vi "GetCtlRefsFromVI.vi"(8 "error in":errorcluster, 11 "VI (Caller)":refnum<vi>) -> (0 "error out":errorcluster, 1 "RefArray":refnum<vi>[](array[refnum]), 2 "RefName Array":string[](array[string]), 3 "VI (Caller) Out":refnum<vi>)   [LabVIEW 2020, in "CtlReferences.lvlib" / "CtlReferences.lvclass"]
uses:
  CtlReferences.lvclass
  TypeDefs/ClassID_Enum.ctl
  CtlReferences.lvclass/CtlReferences.ctl
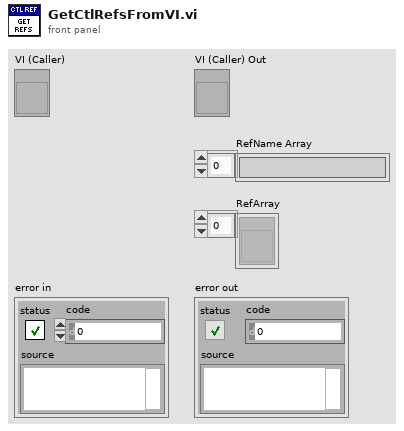
[diagram p1: front panel]
types:
  T1 = typedef "CtlReferences.lvlib/CtlReferences.lvclass/ClassID_Enum.ctl" = enum32{"0 <undefined>", "1 <undefined>", "2 <undefined>", "Generic", "Decoration", "Text", "Control", "ColorBox", "Boolean", "RefNum", "Variant", "Path", "ListBox", "Table", "Array", "Picture", "ActiveXContainer", "Numeric", "Digital", "NamedNumeric", "ColorRamp", "Slide", "GraphOrChart", "WaveformChart", "WaveformGraph", "IntensityChart", "IntensityGraph", "String", "IOName", "ComboBox", "Cluster", "Panel", "Knob", "NumWithScale", "Ring", "Enum", "GObject", "Plot", "Cursor", "NumericText", "Scale", "ColorScale", "GraphScale", "ColorGraphScale", "TypedRefNum", "OldKnobScale", "MCListbox", "MeasureData", "BVTag", "DAQName", "VISAName", "IVIName", "SlideScale", "TabControl", "Page", "TabArrayTabControl", "ConPane"}
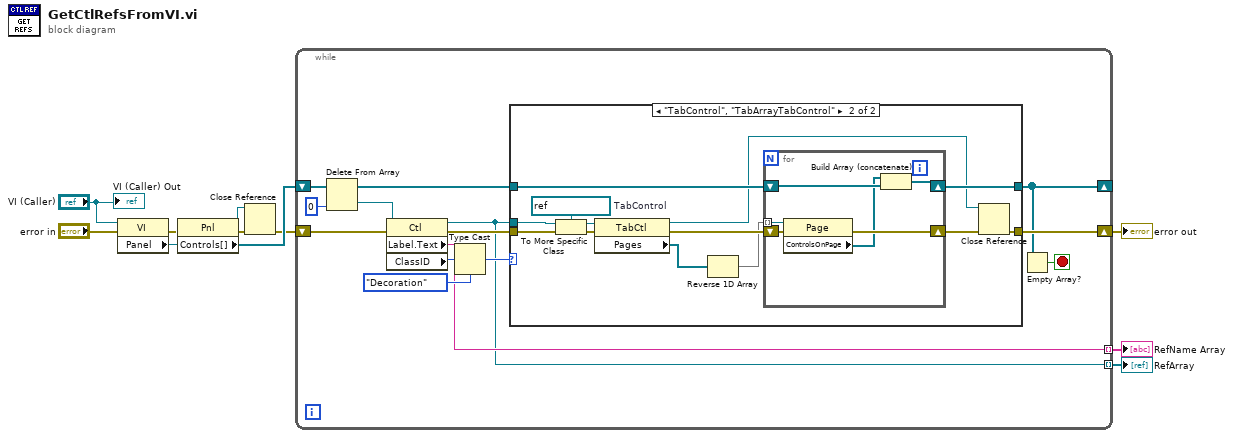
[diagram p0: block diagram]
diagram:
  n1 = property class="VI"(reference="VI (Caller)", error in="error in") -> (error out=w9:errorcluster, "Panel"=w10:refnum<vi>)  [unwired: 1 out]
  n2 = property class="Pnl"(reference=w10, error in=w9) -> (reference out=w6:refnum<vi>, error out=w7:errorcluster, "Controls[]"=w5:refnum<vi>[])
  n3 = Close Reference(reference=w6, error in (no error)=w7) -> (error out=w4:errorcluster)
  n4 = while {
    shift-right: [w21] -> _
    shift-left: w5 -> [w24]
    shift-right: [w25] -> w1
    shift-left: w4 -> [w18]
    tunnel: [w13] -> w3 mode=indexing
    tunnel: [w12] -> w2 mode=indexing
    stop <- w20 stop-if-true
    n5 = Delete From Array(array=w24, index=0) -> (deleted portion=w15:refnum<vi>, array with subset deleted=w22:refnum<vi>[])  [unwired: 1 in]
    n6 = property class="Ctl"(reference=w15, error in=w18) -> (reference out=w12:refnum<vi>, error out=w17:errorcluster, "Label.Text"=w13:string, "ClassID"=w19:u32)
    n7 = Type Cast(type=ClassID_Enum."Decoration" ("ClassID Name"), x=w19) -> (*(type *) &x=w16:T1)
    n8 = case shown="\"TabControl\", \"TabArrayTabControl\"" w16 {
      tunnel: [w26 w40] -> w25
      tunnel: w22 -> [w27 w39]
      tunnel: [w27 w36] -> w21
      tunnel: w12 -> [_ w35]
      tunnel: w17 -> [w26 w30]
      frame Default {
      }
      frame "TabControl", "TabArrayTabControl" {
        w37 = refnum<vi> refnum  # TabControl
        n9 = To More Specific Class(target class=w37, reference=w35, error in=w30) -> (specific class reference=w38:refnum<vi>, error out=w31:errorcluster)
        n10 = property class="TabCtl"(reference=w38, error in=w31) -> (reference out=w33:refnum<vi>, error out=w34:errorcluster, "Pages"=w29:refnum<vi>[])
        n11 = Reverse 1D Array(array=w29) -> (reversed array=w28:refnum<vi>[])
        n12 = for {
          tunnel: w28 -> [w46] mode=indexing
          shift-right: [w44] -> w32
          shift-left: w34 -> [w45]
          shift-right: [w43] -> w36
          shift-left: w39 -> [w42]
          n13 = property class="Page"(reference=w46, error in=w45) -> (error out=w44:errorcluster, "ControlsOnPage"=w41:refnum<vi>[])  [unwired: 1 out]
          n14 = Build Array (concatenate)(w41, w42) -> (w43:refnum<vi>[])
        }
        n15 = Close Reference(reference=w33, error in (no error)=w32) -> (error out=w40:errorcluster)
      }
    }
    n16 = Empty Array?(array=w21) -> (empty?=w20:bool)
  }
  "RefName Array" <- w3
  "RefArray" <- w2
  "error out" <- w1
  "VI (Caller) Out" <- "VI (Caller)"
